vi "CalculateHalfTheta.vi"(11 "cosHalfTheta":dbl) -> (3 "HalfTheta":dbl)   [LabVIEW 2016]
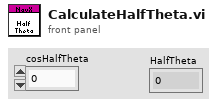
[diagram p1: front panel]
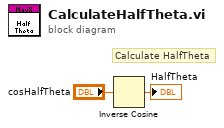
[diagram p0: block diagram]
diagram:
  # "Calculate HalfTheta"
  n1 = Inverse Cosine(1:"cosHalfTheta") -> (0:→"HalfTheta":dbl)
